vi "Tusk.TuskBox.vi"(7 "Operation":T1, 8 "error in (no error)":errorcluster, 10 "Tusk in":refnum<class "Tusk.lvclass">, 11 "Global Name":string) -> (0 "error out":errorcluster, 2 "Tusk out":refnum<class "Tusk.lvclass">)   [LabVIEW 2018, in "Application.lvlib" / "Tusk.lvclass"]
uses:
  Tusk.lvclass
  Controls/Tusk.TuskBoxOperation.ctl
  Dictionary Class/Dictionary.lvclass/Dictionary.ctl
  3ec95ebe-8471-495b-a686-c73d9de2481d.vi
  61460e02-18fd-4935-87ba-760dc3a4827d.vi
  Dictionary Class/VIs/Get Data DVR.vi
  <vilib>/Utility/error.llb/Error Cluster From Error Code.vi
  <vilib>/ErrorRing/Error Ring.xnode
  Dictionary Class/Dictionary.lvclass
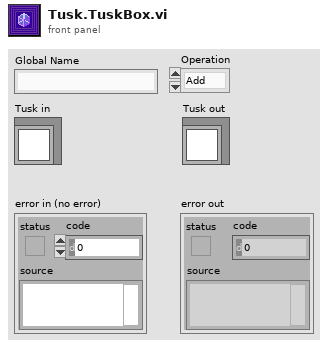
[diagram p1: front panel]
types:
  T1 = typedef "Application.lvlib/Tusk.lvclass/Tusk.TuskBoxOperation.ctl" = enum16{"Add", "Get", "Remove"}
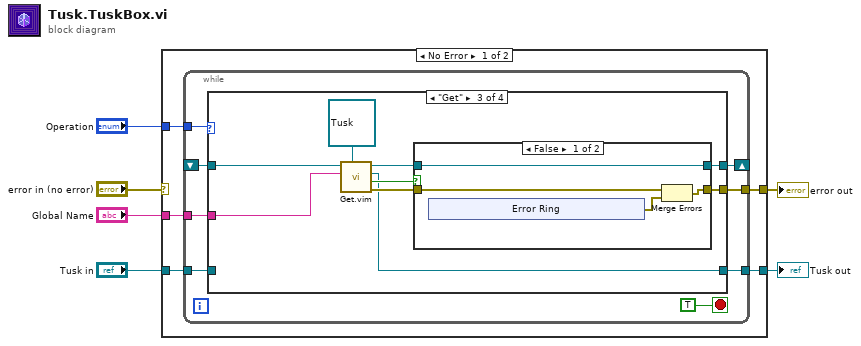
[diagram p0: block diagram]
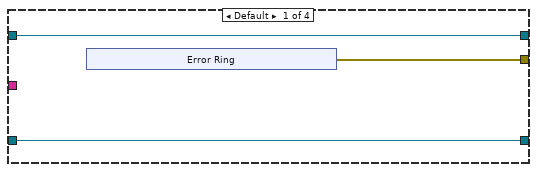
[diagram p2: hidden frame]
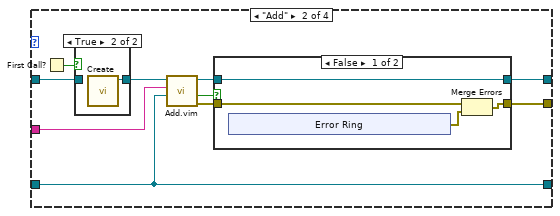
[diagram p3: hidden frame]
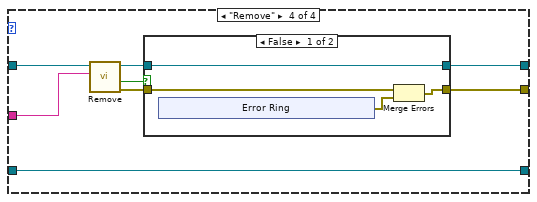
[diagram p7: hidden frame]
diagram:
  n1 = case shown="No Error" "error in (no error)" {
    selector: "error in (no error)" -> [_ w86]
    tunnel: "Operation" -> [w11 _]
    tunnel: "Tusk in" -> [w10 w87]
    tunnel: "Global Name" -> [w9 _]
    tunnel: [w8 w87] -> w3
    tunnel: [w7 w86] -> w2
    frame No Error {
      n2 = while {
        shift-right: [w19] -> _
        shift-left: _ -> [w17]
        tunnel: w11 -> [w18]
        tunnel: [w16] -> w7
        tunnel: w10 -> [w14]
        tunnel: w9 -> [w15]
        tunnel: [w13] -> w8
        stop <- TRUE stop-if-true
        n3 = case shown="\"Get\"" w18 {
          tunnel: [w22 w29 w53 w69] -> w19
          tunnel: w17 -> [w22 w34 w57 w75]
          tunnel: [w20 w28 w51 w71] -> w16
          tunnel: w15 -> [_ w33 w56 w74]
          tunnel: w14 -> [w21 w27 _ w68]
          tunnel: [w21 w27 w49 w68] -> w13
          frame Default {
            n4 = xnode "Error Ring"() -> ("error out"=w20:errorcluster)
          }
          frame "Add" {
            n5 = First Call?() -> (First Call?: T/F=w35:bool)
            n6 = case shown="True" w35 {
              tunnel: [w47 w48] -> w36
              tunnel: w34 -> [w47 _]
              frame False {
              }
              frame True {
                n7 = call "Create.vi"() -> ("Dictionary out"=w48:refnum<class "Dictionary.lvclass">)  [unwired: 10 in, 1 out]
              }
            }
            n8 = call "Add.vim"("Value"=w27, "Key"=w33, "Dictionary in"=w36) -> ("error out"=w32:errorcluster, "Success?"=w31:bool, "Dictionary out"=w30:refnum<class "Dictionary.lvclass">)  [unwired: 6 in]
            n9 = case shown="False" w31 {
              tunnel: w30 -> [w40 w46]
              tunnel: [w40 w46] -> w29
              tunnel: w32 -> [w39 w45]
              tunnel: [w38 w45] -> w28
              frame False {
                n10 = xnode "Error Ring"() -> ("error out"=w37:errorcluster)
                n11 = Merge Errors(w39, w37) -> (w38:errorcluster)
              }
              frame True {
              }
            }
          }
          frame "Get" {
            n12 = call "Get.vim"("Type/Default"=refnum<class "Tusk.lvclass"> refnum ("Tusk in"), "Key"=w56, "Dictionary in"=w57) -> ("error out"=w52:errorcluster, "Found?"=w50:bool, "Value"=w49:refnum<class "Tusk.lvclass">, "Dictionary out"=w54:refnum<class "Dictionary.lvclass">)  [unwired: 5 in]
            n13 = case shown="False" w50 {
              tunnel: w54 -> [w61 w67]
              tunnel: [w61 w67] -> w53
              tunnel: w52 -> [w60 w66]
              tunnel: [w58 w66] -> w51
              frame False {
                n14 = xnode "Error Ring"() -> ("error out"=w59:errorcluster)
                n15 = Merge Errors(w60, w59) -> (w58:errorcluster)
              }
              frame True {
              }
            }
          }
          frame "Remove" {
            n16 = call "Remove.vi"("Key"=w74, "Dictionary in"=w75) -> ("error out"=w72:errorcluster, "Success?"=w73:bool, "Dictionary out"=w70:refnum<class "Dictionary.lvclass">)  [unwired: 7 in]
            n17 = case shown="False" w73 {
              tunnel: w72 -> [w79 w84]
              tunnel: [w77 w84] -> w71
              tunnel: w70 -> [w76 w85]
              tunnel: [w76 w85] -> w69
              frame False {
                n18 = xnode "Error Ring"() -> ("error out"=w78:errorcluster)
                n19 = Merge Errors(w79, w78) -> (w77:errorcluster)
              }
              frame True {
              }
            }
          }
        }
      }
    }
    frame Error {
    }
  }
  "Tusk out" <- w3
  "error out" <- w2
